vi "Begin.vi"(11 "Image Size":T1=enum."320x240") -> (0 "error out":errorcluster)   [LabVIEW 2013]
doc: "Called before other user functions, this VI is expected to open initial I/O refnums, load in file data, and do all program initialization. Notice that the <B>error out</B> terminal is simply used for data flow. Wiring it to other structures or subVIs ensures that this VI runs first."
uses:
  <vilib>/Rock Robotics/WPI/Camera/WPI_CameraImageSize.ctl
  <vilib>/Rock Robotics/WPI/DriverStation/WPI_DriverStationRobotMode2.ctl
  <vilib>/Rock Robotics/WPI/Joystick/WPI_JoystickDeviceEnum.ctl
  <vilib>/Rock Robotics/SystemInterfaces/DIO/FPGA_DIOPWMChannel.ctl
  <vilib>/Rock Robotics/SystemInterfaces/DIO/FPGA_DIORelayChannel.ctl
  <vilib>/Rock Robotics/SystemInterfaces/DIO/FPGA_DIOChannel.ctl
  <vilib>/Rock Robotics/SystemInterfaces/Typedef/FPGA_TypedefDigitalModule.ctl
  <vilib>/Rock Robotics/WPI/Solenoid/WPI_SolenoidChannel.ctl
  <vilib>/Rock Robotics/WPI/Encoder/WPI_EncoderType.ctl
  <vilib>/Rock Robotics/SystemInterfaces/Typedef/FPGA_TypedefAnalogModule.ctl
  <vilib>/Rock Robotics/SystemInterfaces/AI/FPGA_AIChannel.ctl
  RefnameEnum.ctl
  Sally_Dashboard_2014/DBNameEnum.ctl
  <vilib>/Rock Robotics/WPI/Solenoid/WPI_SolenoidValue.ctl
  <vilib>/Rock Robotics/WPI/SafetyOutput/WPI_SafetyOutputConfigMenu.ctl
  QueueInstruction.ctl
  SubsystemEnum.ctl
  ActionEnum.ctl
  TeleopData.ctl
  <vilib>/Rock Robotics/SystemInterfaces/CounterEncoderSourceConvertion/FPGA_CounterEncoderSourceConvertionLVSourceType.ctl
  <vilib>/Rock Robotics/SystemInterfaces/DIO/FPGA_DIODigitalSourceChannel.ctl
  <vilib>/Rock Robotics/SystemInterfaces/AnalogTrigger/FPGA_AnalogTriggerIndex.ctl
  <vilib>/Rock Robotics/SystemInterfaces/AnalogTrigger/FPGA_AnalogTriggerOutType.ctl
  Robot Global Data.vi
  <vilib>/Rock Robotics/WPI/RobotDrive/WPI_RobotDriveOpen2MotorWithTalon.vi
  <vilib>/Rock Robotics/WPI/MotorControl/WPI_MotorControlOpen Talon.vi
  <vilib>/Rock Robotics/WPI/Counter/WPI_CounterDigitalInputToDigitalSource.vi
  <vilib>/Rock Robotics/WPI/Solenoid/WPI_SolenoidOpenSingle.vi
  <vilib>/Rock Robotics/WPI/Solenoid/WPI_SolenoidSetEnum.vi
  <vilib>/Rock Robotics/WPI/MotorControl/WPI_MotorControlOpen Jaguar.vi
  <vilib>/Rock Robotics/WPI/Compressor/WPI_CompressorGetSetRefNum.vi
  <vilib>/Rock Robotics/WPI/Counter/WPI_CounterOpen UpDown Mode.vi
  <vilib>/Rock Robotics/WPI/Camera/WPI_CameraWhite Balance Values.ctl
  <vilib>/Rock Robotics/WPI/Camera/WPI_CameraExposure Values.ctl
  <vilib>/Rock Robotics/WPI/Camera/WPI_CameraFrameRate.ctl
  <vilib>/Rock Robotics/SystemInterfaces/AI/FPGA_AIGyroChannel.ctl
  <vilib>/Rock Robotics/SystemInterfaces/Typedef/FPGA_TypedefAnalogModuleForGyro.ctl
panel:
  in  "LowerLimit (v)":dbl=-1.0
  in  "UpperLimit (v)":dbl=1.0
  out "error out 2":errorcluster
  in  "Version String":string="TruongFramework 1.5.2"
  # "DON'T FORGET TO MAKE THIS DEFAULT"
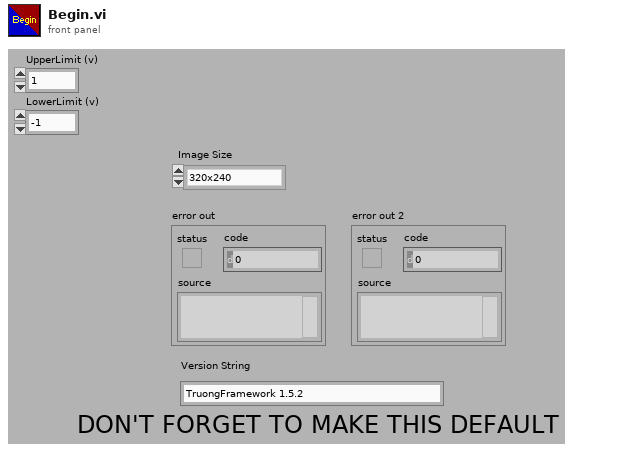
[diagram p1: front panel]
types:
  T1 = typedef "WPI_CameraImageSize.ctl" = enum16{"640x480", "320x240", "160x120"}
  T2 = typedef "TeleopData.ctl" = cluster{"cTankDriveLeft":dbl, "cTankDriveRight":dbl, "cHalfSpeed":bool, "cClimbWeight":bool, "cClimbStart":bool, "cRpmControl":dbl, "cAngleControl":dbl, "cQuickShoot":bool, "cLauncherWheel":bool, "cFirePneumatic":bool, "cPresetLow":bool, "cPresetHigh":bool, "cPresetClimbLow":bool, "cPresetClimbHigh":bool, "cLauncherAngle":bool, "cResetAngleEncoder":bool, "IDNum":i32, "TeleopInterval":i32}
  T3 = typedef "QueueInstruction.ctl" = cluster{"Data":variant, "Subsystem":T4, "Action":T5}
  T4 = typedef "SubsystemEnum.ctl" = enum16{"TankDrive", "FirePneumatic", "Climber", "ClimbWeight", "ShooterAngle"}
  T5 = typedef "ActionEnum.ctl" = enum16{"Init", "SetValue"}
  T6 = typedef "WPI_SafetyOutputConfigMenu.ctl" = enum16{"Enable", "Disable"}
  T7 = typedef "WPI_SolenoidValue.ctl" = enum16{"Off", "On", "Forward", "Reverse"}
  T8 = typedef "RefnameEnum.ctl" = enum16{"FireLauncher", "Climber", "Shield", "TankDrive", "DriveEncoderL", "DriveEncoderR", "LauncherMotorRPM", "LauncherEncoderAnalog", "LauncherEncoderRPM", "ShooterLS", "DriveAlignLSLeft", "DriveAlignLSRight", "ClimbingLS", "LauncherEncoderAngle", "LauncherMotorAngle", "Gamepad1", "Gamepad2", "Compressor", "ClimbWeightSol3", "ClimbWeightSol4"}
  T9 = typedef "WPI_SolenoidChannel.ctl" = enum8{"Solenoid 1", "Solenoid 2", "Solenoid 3", "Solenoid 4", "Solenoid 5", "Solenoid 6", "Solenoid 7", "Solenoid 8", "Invalid"}
  T10 = typedef "FPGA_DIOChannel.ctl" = enum8{"DIO 1", "DIO 2", "DIO 3", "DIO 4", "DIO 5", "DIO 6", "DIO 7", "DIO 8", "DIO 9", "DIO 10", "DIO 11", "DIO 12", "DIO 13", "DIO 14", "Invalid"}
  T11 = typedef "FPGA_TypedefDigitalModule.ctl" = enum16{"Digital Module 1", "Digital Module 2"}
  T12 = typedef "DBNameEnum.ctl" = enum16{"AutoInstructions", "DriveLoopTime", "DriveAlignLSLeft", "DriveAlignLSRight", "Use2DriveAlign", "ClimbLS", "LauncherAngleMatches", "FrameworkVersion", "sLauncherAngle", "LauncherTargetAngle", "sLauncherRPM", "LauncherTargetRPM", "sDriveDistance", "LauncherMotorValue", "PullbackTol", "FireTol", "LauncherRPMTol", "LauncherAngleTol", "InitialWait", "WaitBetweenLaunch", "AnglePresets", "RPMPresets", "UseAngleEncoder", "UseLauncherEncoder", "UseLauncherPID", "QSWaitBeforeFire", "QSWaitBeforeRetract", "AngleForwardValue", "AngleBackwardValue", "UseClusterArray", "BackupAuto", "ReverseDriveIndicate", "HalfSpeedFactor"}
  T13 = typedef "FPGA_AIChannel.ctl" = enum8{"AI 1", "AI 2", "AI 3", "AI 4", "AI 5", "AI 6", "AI 7", "AI 8", "Invalid"}
  T14 = typedef "FPGA_TypedefAnalogModule.ctl" = enum16{"Analog Module 1", "Analog Module 2"}
  T15 = typedef "WPI_EncoderType.ctl" = enum16{"1x", "2x", "4x"}
  T16 = typedef "FPGA_DIORelayChannel.ctl" = enum8{"Relay 1", "Relay 2", "Relay 3", "Relay 4", "Relay 5", "Relay 6", "Relay 7", "Relay 8", "Invalid"}
  T17 = typedef "FPGA_DIOPWMChannel.ctl" = enum8{"PWM 1", "PWM 2", "PWM 3", "PWM 4", "PWM 5", "PWM 6", "PWM 7", "PWM 8", "PWM 9", "PWM 10", "Invalid"}
  T18 = typedef "WPI_JoystickDeviceEnum.ctl" = enum16{"USB 1", "USB 2", "USB 3", "USB 4", "Kinect 1", "Kinect 2"}
  T19 = typedef "WPI_DriverStationRobotMode2.ctl" = enum16{"Autonomous Disabled", "Autonomous Enabled", "Teleop Disabled", "Teleop Enabled", "Timeout", "Finish", "Test Disabled", "Test Enabled"}
  T20 = enum16{"Rising Edge", "Falling Edge", "Raising & Falling Edge", "Disabled"}
  T21 = typedef "WPI_DigitalInputDevRef.ctl" = cluster{"DevStatus":errorcluster, "DIO Channel":T10, "Digital Module":T11}
  T22 = typedef "FPGA_CounterEncoderSourceConvertionLVSourceType.ctl" = cluster{"DevStatus":errorcluster, "AnalogTriggerMode?":bool, "DigitalMode":cluster{"Digital Module":T11, "DIO Channel":T23}, "AnalogTriggerMode":cluster{"AnalogTriggerIndex":T24, "OutputType":T25}}
  T23 = typedef "FPGA_DIODigitalSourceChannel.ctl" = enum8{"DIO 1", "DIO 2", "DIO 3", "DIO 4", "DIO 5", "DIO 6", "DIO 7", "DIO 8", "DIO 9", "DIO 10", "DIO 11", "DIO 12", "DIO 13", "DIO 14", "Disabled"}
  T24 = typedef "FPGA_AnalogTriggerIndex.ctl" = enum8{"Trig 0", "Trig 1", "Trig 2", "Trig 3", "Trig 4", "Trig 5", "Trig 6", "Trig 7", "Invalid"}
  T25 = typedef "FPGA_AnalogTriggerOutType.ctl" = enum16{"InWindow", "TriggerState", "Rising", "Falling"}
  T26 = typedef "WPI_EncoderDevRef.ctl" = cluster{"DevStatus":errorcluster, "EncoderIndex":T27, "CounterIndex":T28, "DistancePerCount":dbl, "Decoding Type":T15}
  T27 = typedef "FPGA_EncoderIdx.ctl" = enum8{"Enc 0", "Enc 1", "Enc 2", "Enc 3", "Invalid"}
  T28 = typedef "FPGA_CounterCtrSystemIndex.ctl" = enum8{"Ctr 0", "Ctr 1", "Ctr 2", "Ctr 3", "Ctr 4", "Ctr 5", "Ctr 6", "Ctr 7", "Invalid"}
  T29 = typedef "WPI_CounterDevRef.ctl" = cluster{"DevStatus":errorcluster, "CntIndex":T28}
  T30 = typedef "FPGA_AIGyroChannel.ctl" = enum8{"AI 1", "AI 2", "Invalid"}
  T31 = typedef "FPGA_TypedefAnalogModuleForGyro.ctl" = enum16{"Analog Module 1"}
  T32 = typedef "WPI_GyroDevRef.ctl" = cluster{"DevStatus":errorcluster, "Analog Module":T14, "Analog Channel":T13, "Offset":dbl, "Gain (VoltsPerDegree/Second)":dbl}
  T33 = typedef "WPI_MotorControlDeviceRef.ctl" = cluster{"DeviceStatus":errorcluster, "Type":enum16{"PWM", "CAN"}, "PWM":cluster{"Digital Module":T11, "PWM Channel":T17, "DeadBand":T34}, "CAN":cluster{"Device Number":u8, "Control Mode":T35, "Semaphore":T36, "Max Vout":dbl}, "Invert":bool, "TransformRef":T37, "InvTransformRef":T37}
  T34 = typedef "WPI_PWMDeadband.ctl" = cluster{"Name":string, "maxPositivePwm":i32, "minPositivePwm":i32, "centerPwm":i32, "maxNegativePwm":i32, "minNegativePwm":i32, "angularRange":u16}
  T35 = typedef "WPI_CANJaguar_ControlMode.ctl" = enum8{"Percent VBus", "Current", "Speed", "Position", "Voltage"}
  T36 = typedef "Semaphore RefNum" = refnum<k1>
  T37 = typedef "WPI_PWMTransform_ConPane.ctl" = refnum<vi>
  T38 = typedef "WPI_RelayDevRef.ctl" = cluster{"DevStatus":errorcluster, "Relay Channel":T16, "Digital Module":T11, "Relay Direction":T39}
  T39 = typedef "WPI_RelayDirection.ctl" = enum16{"Both directions", "Forward only", "Reverse only"}
  T40 = typedef "WPI_SolenoidDevRef.ctl" = cluster{"DevStatus":errorcluster, "Solenoid Module":T41, "Forward Solenoid Channel":T9, "Reverse Solenoid Channel":T9}
  T41 = typedef "FPGA_TypedefSolenoidModule.ctl" = enum16{"Solenoid Module 1", "Solenoid Module 2"}
  T42 = typedef "WPI_CompressorDevRef.ctl" = cluster{"DevStatus":errorcluster, "DigitalInputDevRef":T21, "RelayDevRef":T38}
  T43 = typedef "WPI_RobotDriveDevRef.ctl" = cluster{"DevStatus":errorcluster, "Motors[]":T33[], "Square Inputs":bool, "Max Output":dbl, "Isochronous":bool}
  T44 = typedef "WPI_CameraFrameRate.ctl" = u32
  T45 = typedef "WPI_CameraExposure Values.ctl" = enum16{"Auto", "Flicker-free 50 Hz", "Flicker-free 60 Hz", "Hold current"}
  T46 = typedef "WPI_CameraWhite Balance Values.ctl" = enum16{"Auto", "Fixed indoor", "Fixed outdoor 1", "Fixed outdoor 2", "Fixed fluorescent 1", "Fixed fluorescent 2", "Hold current"}
  T47 = typedef "WPI_CameraDevRef.ctl" = cluster{"Camera Address":string, "CameraStatus":errorcluster, "Acquire Image Notifier":refnum<notifier>}
  T48 = typedef "WPI_JoystickDevRef.ctl" = cluster{"Device":T18}
  T49 = typedef "WPI_AnalogChannelDevRef.ctl" = cluster{"DevStatus":errorcluster, "Analog Module":T14, "Analog Channel":T13}
  T50 = typedef "FPGA_AnalogTriggerDevRef.ctl" = cluster{"DevStatus":errorcluster, "AnalogTriggerIndex":T24}
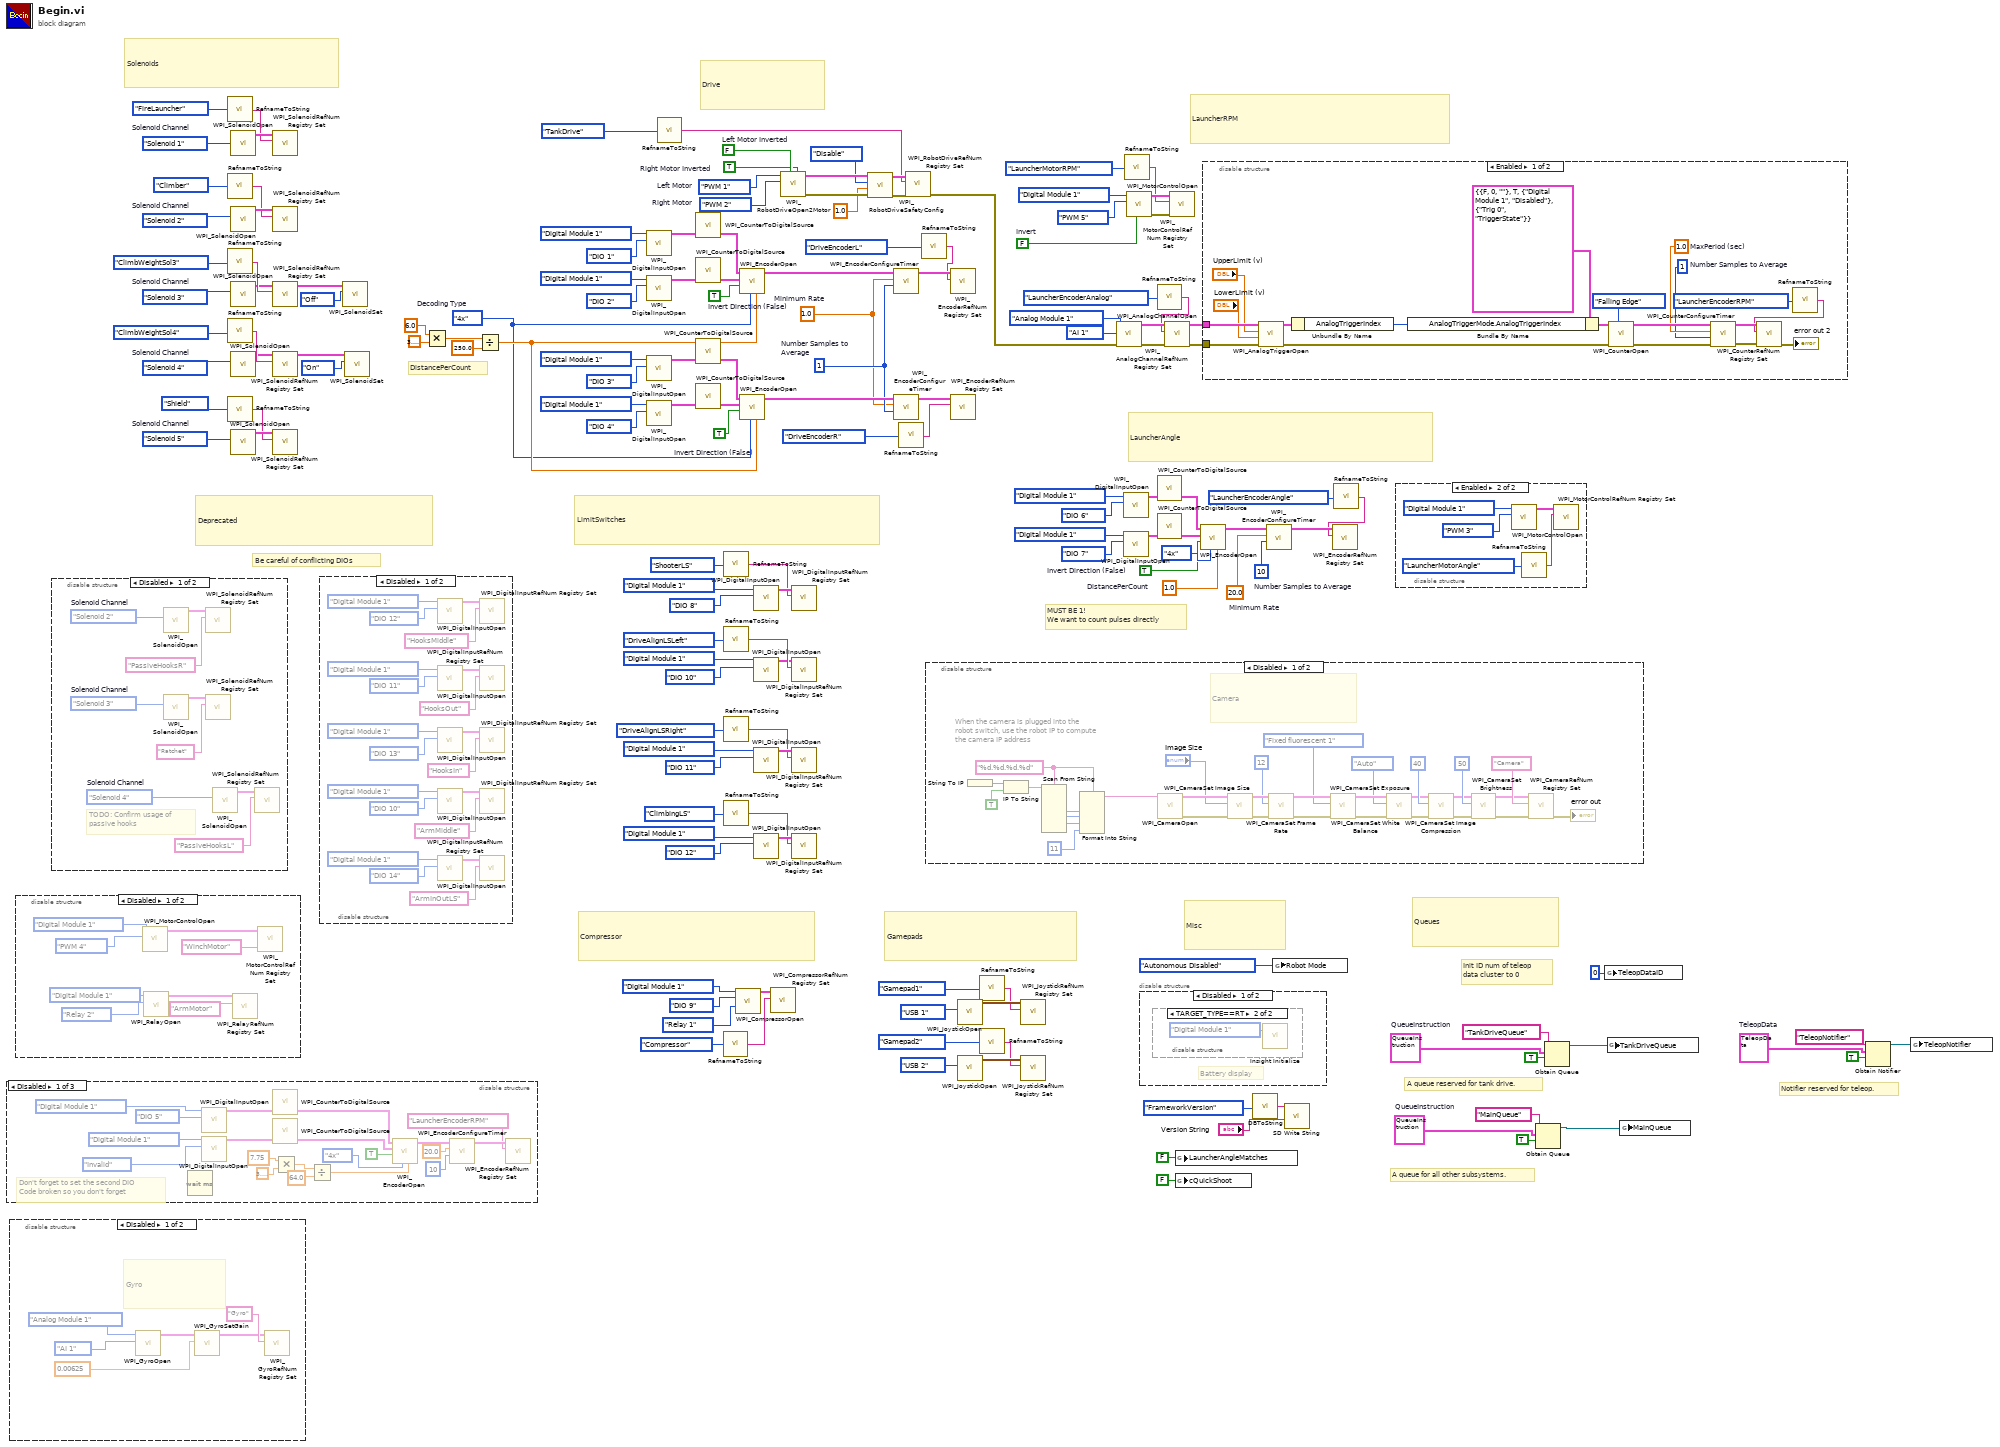
[diagram p0: block diagram]
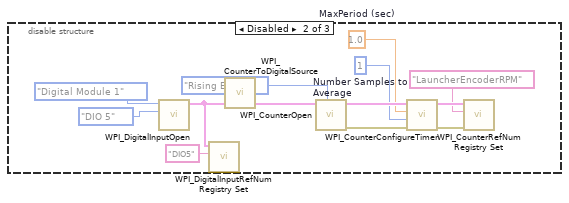
[diagram p8: hidden frame]
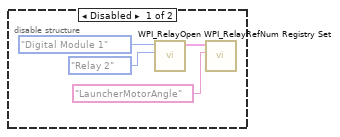
[diagram p12: hidden frame]
diagram:
  w5 = T2 {"cTankDriveLeft"=0.0, "cTankDriveRight"=0.0, "cHalfSpeed"=FALSE, "cClimbWeight"=FALSE, "cClimbStart"=FALSE, "cRpmControl"=0.0, "cAngleControl"=0.0, "cQuickShoot"=FALSE, "cLauncherWheel"=FALSE, "cFirePneumatic"=FALSE, "cPresetLow"=FALSE, "cPresetHigh"=FALSE, "cPresetClimbLow"=FALSE, "cPresetClimbHigh"=FALSE, "cLauncherAngle"=FALSE, "cResetAngleEncoder"=FALSE, "IDNum"=0, "TeleopInterval"=0}  # TeleopData
  w10 = T3 {"Data"=variant, "Subsystem"=enum."TankDrive", "Action"=enum."Init"}  # QueueInstruction
  w11 = T3 {"Data"=variant, "Subsystem"=enum."TankDrive", "Action"=enum."Init"}  # QueueInstruction
  w25 = WPI_SolenoidChannel."Solenoid 4"  # Solenoid Channel
  w29 = WPI_SolenoidChannel."Solenoid 3"  # Solenoid Channel
  w85 = 1.0  # DistancePerCount
  w88 = TRUE  # Invert Direction (False)
  w89 = TRUE  # Invert Direction (False)
  w93 = WPI_SolenoidChannel."Solenoid 5"  # Solenoid Channel
  w95 = WPI_SolenoidChannel."Solenoid 2"  # Solenoid Channel
  w100 = TRUE  # Invert Direction (False)
  w102 = u8 10  # Number Samples to Average
  w103 = 20.0  # Minimum Rate
  w115 = WPI_SolenoidChannel."Solenoid 1"  # Solenoid Channel
  w90 = WPI_EncoderType."4x"  # Decoding Type
  w87 = u8 1  # Number Samples to Average
  w86 = 1.0  # Minimum Rate
  w144 = FALSE  # Invert
  w148 = FPGA_DIOPWMChannel."PWM 2"  # Right Motor
  w149 = FPGA_DIOPWMChannel."PWM 1"  # Left Motor
  w150 = TRUE  # Right Motor Inverted
  w151 = FALSE  # Left Motor Inverted
  # "Init ID num of teleop\ndata cluster to 0"
  # "Notifier reserved for teleop."
  # "A queue reserved for tank drive."
  # "A queue for all other subsystems."
  # "Queues"
  # "Be careful of conflicting DIOs"
  # "DistancePerCount"
  # "Deprecated"
  # "LimitSwitches"
  # "Compressor"
  # "Solenoids"
  # "LauncherAngle"
  # "LauncherRPM"
  # "Misc"
  # "Gamepads"
  # "Drive"
  # "MUST BE 1!\nWe want to count pulses directly"
  n1 = disable-structure shown="Disabled" {
    frame Disabled {
      # "Don't forget to set the second DIO\nCode broken so you don't forget"
      n2 = Wait (ms)() -> ()  [unwired: 1 in, 1 out]
      n3 = call <vilib>:"WPI_DigitalInputOpen.vi"("DIO Channel"=FPGA_DIOChannel."DIO 5", "Digital Module (Module 1)"=FPGA_TypedefDigitalModule."Digital Module 1") -> ("DigitalInputDevRef"=w174:T21)  [unwired: 1 in, 8 out]
      n4 = call <vilib>:"WPI_DigitalInputOpen.vi"("DIO Channel"=FPGA_DIOChannel."Invalid", "Digital Module (Module 1)"=FPGA_TypedefDigitalModule."Digital Module 1") -> ("DigitalInputDevRef"=w175:T21)  [unwired: 1 in, 8 out]
      n5 = call-poly <vilib>:"WPI_CounterToDigitalSource.vi"("DigitalInputDevRef"=w174) -> ("Digital Source"=w173:T22)  [unwired: 6 out]
      n6 = call-poly <vilib>:"WPI_CounterToDigitalSource.vi"("DigitalInputDevRef"=w175) -> ("Digital Source"=w176:T22)  [unwired: 6 out]
      n7 = Multiply(x=7.75, y=3.141592653589793) -> (x*y=w158:dbl)
      n8 = Divide(x=w158, y=64.0) -> (x/y=w161:dbl)
      n9 = call <vilib>:"WPI_EncoderOpen.vi"("DistancePerCount"=w161, "Decoding Type"=WPI_EncoderType."4x", "Invert Direction (False)"=TRUE, "BSource"=w176, "ASource"=w173) -> ("EncoderDevRef"=w170:T26)  [unwired: 3 in, 3 out]
      n10 = call <vilib>:"WPI_EncoderConfigureTimer.vi"("Number Samples to Average"=u8 10, "Minimum Rate"=20.0, "EncoderDevRef"=w170) -> ("EncoderDevRef"=w167:T26)  [unwired: 1 in, 7 out]
      n11 = call <vilib>:"WPI_EncoderRefNum Registry Set.vi"("refnum name"="LauncherEncoderRPM", "EncoderDevRef"=w167) -> ()  [unwired: 8 in, 2 out]
    }
    frame Disabled {
      w187 = u8 1  # Number Samples to Average
      w188 = 1.0  # MaxPeriod (sec)
      n12 = call <vilib>:"WPI_DigitalInputOpen.vi"("DIO Channel"=FPGA_DIOChannel."DIO 5", "Digital Module (Module 1)"=FPGA_TypedefDigitalModule."Digital Module 1") -> ("DigitalInputDevRef"=w178:T21)  [unwired: 8 in, 1 out]
      n13 = call <vilib>:"WPI_DigitalInputRefNum Registry Set.vi"("refnum name"="DIO5", "DigitalInputDevRef"=w178) -> ()  [unwired: 8 in, 2 out]
      n14 = call-poly <vilib>:"WPI_CounterToDigitalSource.vi"("DigitalInputDevRef"=w178) -> ("Digital Source"=w181:T22)  [unwired: 6 out]
      n15 = call-poly <vilib>:"WPI_CounterOpen.vi"("UpEdge"=T20."Rising Edge", "Up Source"=w181) -> ("error out"=w183:errorcluster, "CounterDevRef"=w189:T29)  [unwired: 8 in]
      n16 = call <vilib>:"WPI_CounterConfigureTimer.vi"("error in (no error)"=w183, "Number Samples to Average"=w187, "MaxPeriod (sec)"=w188, "CounterDevRef in"=w189) -> ("error out"=w182:errorcluster, "CounterDevRef out"=w186:T29)  [unwired: 6 in]
      n17 = call <vilib>:"WPI_CounterRefNum Registry Set.vi"("error in (no error)"=w182, "refnum name"="LauncherEncoderRPM", "CounterDevRef"=w186) -> ()  [unwired: 7 in, 2 out]
    }
    frame Enabled {
      # "LauncherRPM Deprecated"
    }
  }
  n18 = disable-structure shown="Disabled" {
    frame Disabled {
      # "Gyro"
      n19 = call <vilib>:"WPI_GyroOpen.vi"("Analog Channel"=FPGA_AIGyroChannel."AI 1", "Analog Module (Module 1)"=FPGA_TypedefAnalogModuleForGyro."Analog Module 1") -> ("GyroDevRef"=w192:T32)  [unwired: 7 in, 2 out]
      n20 = call <vilib>:"WPI_GyroSetGain.vi"("Gain (VoltsPerDegree/Second)"=0.00625, "GyroDevRef"=w192) -> ("GyroDevRef"=w191:T32)  [unwired: 8 in, 1 out]
      n21 = call <vilib>:"WPI_GyroRefNum Registry Set.vi"("refnum name"="Gyro", "GyroDevRef"=w191) -> ()  [unwired: 8 in, 2 out]
    }
    frame Enabled {
    }
  }
  n22 = disable-structure shown="Disabled" {
    frame Disabled {
      n23 = call-poly <vilib>:"WPI_MotorControlOpen.vi"("PWM Channel"=FPGA_DIOPWMChannel."PWM 4", "Digital Module (Module 1)"=FPGA_TypedefDigitalModule."Digital Module 1") -> ("MotorControlDeviceRef"=w201:T33)  [unwired: 8 in, 1 out]
      n24 = call <vilib>:"WPI_RelayOpen.vi"("Relay Channel"=FPGA_DIORelayChannel."Relay 2", "Digital Module (Module 1)"=FPGA_TypedefDigitalModule."Digital Module 1") -> ("RelayDevRef"=w197:T38)  [unwired: 8 in, 1 out]
      n25 = call <vilib>:"WPI_RelayRefNum Registry Set.vi"("refnum name"="ArmMotor", "RelayDevRef"=w197) -> ()  [unwired: 8 in, 2 out]
      n26 = call <vilib>:"WPI_MotorControlRefNum Registry Set.vi"("refnum name"="WinchMotor", "MotorControlDevRef"=w201) -> ()  [unwired: 8 in, 2 out]
    }
    frame Enabled {
    }
  }
  n27 = disable-structure shown="Disabled" {
    frame Disabled {
      w206 = WPI_SolenoidChannel."Solenoid 2"  # Solenoid Channel
      w209 = WPI_SolenoidChannel."Solenoid 4"  # Solenoid Channel
      w212 = WPI_SolenoidChannel."Solenoid 3"  # Solenoid Channel
      # "TODO: Confirm usage of\npassive hooks"
      n28 = call-poly <vilib>:"WPI_SolenoidOpen.vi"("Solenoid Channel"=w206) -> ("SolenoidDevRef"=w205:T40)  [unwired: 2 in, 8 out]
      n29 = call-poly <vilib>:"WPI_SolenoidOpen.vi"("Solenoid Channel"=w212) -> ("SolenoidDevRef"=w211:T40)  [unwired: 2 in, 8 out]
      n30 = call <vilib>:"WPI_SolenoidRefNum Registry Set.vi"("refnum name"="PassiveHooksR", "SolenoidDevRef"=w205) -> ()  [unwired: 8 in, 2 out]
      n31 = call <vilib>:"WPI_SolenoidRefNum Registry Set.vi"("refnum name"="Ratchet", "SolenoidDevRef"=w211) -> ()  [unwired: 8 in, 2 out]
      n32 = call-poly <vilib>:"WPI_SolenoidOpen.vi"("Solenoid Channel"=w209) -> ("SolenoidDevRef"=w208:T40)  [unwired: 2 in, 8 out]
      n33 = call <vilib>:"WPI_SolenoidRefNum Registry Set.vi"("refnum name"="PassiveHooksL", "SolenoidDevRef"=w208) -> ()  [unwired: 8 in, 2 out]
    }
    frame Enabled {
    }
  }
  n34 = call "RefnameToString.vi"("Enum"=RefnameEnum."FireLauncher") -> ("Refname"=w68:string)
  n35 = call "RefnameToString.vi"("Enum"=RefnameEnum."Climber") -> ("Refname"=w66:string)
  n36 = call "RefnameToString.vi"("Enum"=RefnameEnum."ClimbWeightSol3") -> ("Refname"=w32:string)
  n37 = call "RefnameToString.vi"("Enum"=RefnameEnum."ClimbWeightSol4") -> ("Refname"=w28:string)
  n38 = call "RefnameToString.vi"("Enum"=RefnameEnum."Shield") -> ("Refname"=w64:string)
  n39 = call-poly <vilib>:"WPI_SolenoidOpen.vi"("Solenoid Channel"=w115) -> ("SolenoidDevRef"=w114:T40)  [unwired: 2 in, 8 out]
  n40 = call-poly <vilib>:"WPI_SolenoidOpen.vi"("Solenoid Channel"=w95) -> ("SolenoidDevRef"=w94:T40)  [unwired: 2 in, 8 out]
  n41 = call-poly <vilib>:"WPI_SolenoidOpen.vi"("Solenoid Channel"=w29) -> ("SolenoidDevRef"=w30:T40)  [unwired: 2 in, 8 out]
  n42 = call-poly <vilib>:"WPI_SolenoidOpen.vi"("Solenoid Channel"=w25) -> ("SolenoidDevRef"=w26:T40)  [unwired: 2 in, 8 out]
  n43 = call-poly <vilib>:"WPI_SolenoidOpen.vi"("Solenoid Channel"=w93) -> ("SolenoidDevRef"=w92:T40)  [unwired: 2 in, 8 out]
  n44 = call <vilib>:"WPI_SolenoidRefNum Registry Set.vi"("refnum name"=w68, "SolenoidDevRef"=w114) -> ()  [unwired: 8 in, 2 out]
  n45 = call <vilib>:"WPI_SolenoidRefNum Registry Set.vi"("refnum name"=w66, "SolenoidDevRef"=w94) -> ()  [unwired: 8 in, 2 out]
  n46 = call <vilib>:"WPI_SolenoidRefNum Registry Set.vi"("refnum name"=w32, "SolenoidDevRef"=w30) -> ("SolenoidDevRef"=w24:T40)  [unwired: 8 in, 1 out]
  n47 = call <vilib>:"WPI_SolenoidRefNum Registry Set.vi"("refnum name"=w28, "SolenoidDevRef"=w26) -> ("SolenoidDevRef"=w23:T40)  [unwired: 8 in, 1 out]
  n48 = call <vilib>:"WPI_SolenoidRefNum Registry Set.vi"("refnum name"=w64, "SolenoidDevRef"=w92) -> ()  [unwired: 8 in, 2 out]
  n49 = disable-structure shown="Disabled" {
    frame Disabled {
      n50 = call <vilib>:"WPI_DigitalInputOpen.vi"("DIO Channel"=FPGA_DIOChannel."DIO 12", "Digital Module (Module 1)"=FPGA_TypedefDigitalModule."Digital Module 1") -> ("DigitalInputDevRef"=w216:T21)  [unwired: 8 in, 1 out]
      n51 = call <vilib>:"WPI_DigitalInputOpen.vi"("DIO Channel"=FPGA_DIOChannel."DIO 11", "Digital Module (Module 1)"=FPGA_TypedefDigitalModule."Digital Module 1") -> ("DigitalInputDevRef"=w220:T21)  [unwired: 8 in, 1 out]
      n52 = call <vilib>:"WPI_DigitalInputOpen.vi"("DIO Channel"=FPGA_DIOChannel."DIO 13", "Digital Module (Module 1)"=FPGA_TypedefDigitalModule."Digital Module 1") -> ("DigitalInputDevRef"=w224:T21)  [unwired: 8 in, 1 out]
      n53 = call <vilib>:"WPI_DigitalInputOpen.vi"("DIO Channel"=FPGA_DIOChannel."DIO 10", "Digital Module (Module 1)"=FPGA_TypedefDigitalModule."Digital Module 1") -> ("DigitalInputDevRef"=w228:T21)  [unwired: 8 in, 1 out]
      n54 = call <vilib>:"WPI_DigitalInputOpen.vi"("DIO Channel"=FPGA_DIOChannel."DIO 14", "Digital Module (Module 1)"=FPGA_TypedefDigitalModule."Digital Module 1") -> ("DigitalInputDevRef"=w232:T21)  [unwired: 8 in, 1 out]
      n55 = call <vilib>:"WPI_DigitalInputRefNum Registry Set.vi"("refnum name"="HooksMiddle", "DigitalInputDevRef"=w216) -> ()  [unwired: 8 in, 2 out]
      n56 = call <vilib>:"WPI_DigitalInputRefNum Registry Set.vi"("refnum name"="HooksOut", "DigitalInputDevRef"=w220) -> ()  [unwired: 8 in, 2 out]
      n57 = call <vilib>:"WPI_DigitalInputRefNum Registry Set.vi"("refnum name"="HooksIn", "DigitalInputDevRef"=w224) -> ()  [unwired: 8 in, 2 out]
      n58 = call <vilib>:"WPI_DigitalInputRefNum Registry Set.vi"("refnum name"="ArmMiddle", "DigitalInputDevRef"=w228) -> ()  [unwired: 8 in, 2 out]
      n59 = call <vilib>:"WPI_DigitalInputRefNum Registry Set.vi"("refnum name"="ArmInOutLS", "DigitalInputDevRef"=w232) -> ()  [unwired: 8 in, 2 out]
    }
    frame Enabled {
    }
  }
  n60 = call-poly <vilib>:"WPI_SolenoidSet.vi"("Value"=WPI_SolenoidValue."Off", "SolenoidDevRef"=w24) -> ()  [unwired: 8 in, 2 out]
  n61 = call-poly <vilib>:"WPI_SolenoidSet.vi"("Value"=WPI_SolenoidValue."On", "SolenoidDevRef"=w23) -> ()  [unwired: 8 in, 2 out]
  n62 = Multiply(x=6.0, y=3.141592653589793) -> (x*y=w97:dbl)
  n63 = Divide(x=w97, y=250.0) -> (x/y=w91:dbl)
  n64 = call <vilib>:"WPI_DigitalInputOpen.vi"("DIO Channel"=FPGA_DIOChannel."DIO 1", "Digital Module (Module 1)"=FPGA_TypedefDigitalModule."Digital Module 1") -> ("DigitalInputDevRef"=w136:T21)  [unwired: 1 in, 8 out]
  n65 = call <vilib>:"WPI_DigitalInputOpen.vi"("DIO Channel"=FPGA_DIOChannel."DIO 2", "Digital Module (Module 1)"=FPGA_TypedefDigitalModule."Digital Module 1") -> ("DigitalInputDevRef"=w137:T21)  [unwired: 1 in, 8 out]
  n66 = call <vilib>:"WPI_DigitalInputOpen.vi"("DIO Channel"=FPGA_DIOChannel."DIO 3", "Digital Module (Module 1)"=FPGA_TypedefDigitalModule."Digital Module 1") -> ("DigitalInputDevRef"=w123:T21)  [unwired: 1 in, 8 out]
  n67 = call <vilib>:"WPI_DigitalInputOpen.vi"("DIO Channel"=FPGA_DIOChannel."DIO 4", "Digital Module (Module 1)"=FPGA_TypedefDigitalModule."Digital Module 1") -> ("DigitalInputDevRef"=w124:T21)  [unwired: 1 in, 8 out]
  n68 = call "RefnameToString.vi"("Enum"=RefnameEnum."TankDrive") -> ("Refname"=w16:string)
  n69 = call-poly <vilib>:"WPI_CounterToDigitalSource.vi"("DigitalInputDevRef"=w136) -> ("Digital Source"=w135:T22)  [unwired: 6 out]
  n70 = call-poly <vilib>:"WPI_CounterToDigitalSource.vi"("DigitalInputDevRef"=w137) -> ("Digital Source"=w138:T22)  [unwired: 6 out]
  n71 = call-poly <vilib>:"WPI_CounterToDigitalSource.vi"("DigitalInputDevRef"=w123) -> ("Digital Source"=w122:T22)  [unwired: 6 out]
  n72 = call-poly <vilib>:"WPI_CounterToDigitalSource.vi"("DigitalInputDevRef"=w124) -> ("Digital Source"=w125:T22)  [unwired: 6 out]
  n73 = call "RefnameToString.vi"("Enum"=RefnameEnum."Compressor") -> ("Refname"=w45:string)
  n74 = call "RefnameToString.vi"("Enum"=RefnameEnum."ShooterLS") -> ("Refname"=w51:string)
  n75 = call "RefnameToString.vi"("Enum"=RefnameEnum."DriveAlignLSLeft") -> ("Refname"=w38:string)
  n76 = call "RefnameToString.vi"("Enum"=RefnameEnum."DriveAlignLSRight") -> ("Refname"=w49:string)
  n77 = call "RefnameToString.vi"("Enum"=RefnameEnum."ClimbingLS") -> ("Refname"=w47:string)
  n78 = call <vilib>:"WPI_CompressorOpen.vi"("Pressure Switch Digital Module (Module 1)"=FPGA_TypedefDigitalModule."Digital Module 1" ("Pressure Switch\nand Relay Module"), "Pressure Switch DIO Channel"=FPGA_DIOChannel."DIO 9" ("Pressure Switch Channel"), "Relay Channel"=FPGA_DIORelayChannel."Relay 1") -> ("CompressorDevRef"=w139:T42)  [unwired: 2 in, 10 out]
  n79 = call <vilib>:"WPI_EncoderOpen.vi"("DistancePerCount"=w91, "Decoding Type"=w90, "Invert Direction (False)"=w89, "BSource"=w138, "ASource"=w135) -> ("EncoderDevRef"=w132:T26)  [unwired: 3 in, 3 out]
  n80 = call <vilib>:"WPI_EncoderOpen.vi"("DistancePerCount"=w91, "Decoding Type"=w90, "Invert Direction (False)"=w88, "BSource"=w125, "ASource"=w122) -> ("EncoderDevRef"=w119:T26)  [unwired: 3 in, 3 out]
  n81 = call <vilib>:"WPI_DigitalInputOpen.vi"("DIO Channel"=FPGA_DIOChannel."DIO 8", "Digital Module (Module 1)"=FPGA_TypedefDigitalModule."Digital Module 1") -> ("DigitalInputDevRef"=w128:T21)  [unwired: 8 in, 1 out]
  n82 = call <vilib>:"WPI_DigitalInputOpen.vi"("DIO Channel"=FPGA_DIOChannel."DIO 10", "Digital Module (Module 1)"=FPGA_TypedefDigitalModule."Digital Module 1") -> ("DigitalInputDevRef"=w34:T21)  [unwired: 8 in, 1 out]
  n83 = call <vilib>:"WPI_DigitalInputOpen.vi"("DIO Channel"=FPGA_DIOChannel."DIO 11", "Digital Module (Module 1)"=FPGA_TypedefDigitalModule."Digital Module 1") -> ("DigitalInputDevRef"=w78:T21)  [unwired: 8 in, 1 out]
  n84 = call <vilib>:"WPI_DigitalInputOpen.vi"("DIO Channel"=FPGA_DIOChannel."DIO 12", "Digital Module (Module 1)"=FPGA_TypedefDigitalModule."Digital Module 1") -> ("DigitalInputDevRef"=w72:T21)  [unwired: 8 in, 1 out]
  n85 = call <vilib>:"WPI_CompressorRefNum Registry Set.vi"("refnum name"=w45, "CompressorDevRef"=w139) -> ()  [unwired: 8 in, 2 out]
  n86 = call-poly <vilib>:"WPI_RobotDriveOpen2Motor.vi"("Right Motor Inverted"=w150, "Left Motor Inverted"=w151, "Right Motor"=w148, "Left Motor"=w149) -> ("error out"=w17:errorcluster, "RobotDriveDevRef"=w20:T43)  [unwired: 6 in]
  n87 = call <vilib>:"WPI_DigitalInputRefNum Registry Set.vi"("refnum name"=w51, "DigitalInputDevRef"=w128) -> ()  [unwired: 8 in, 2 out]
  n88 = call <vilib>:"WPI_DigitalInputRefNum Registry Set.vi"("refnum name"=w38, "DigitalInputDevRef"=w34) -> ()  [unwired: 8 in, 2 out]
  n89 = call <vilib>:"WPI_DigitalInputRefNum Registry Set.vi"("refnum name"=w49, "DigitalInputDevRef"=w78) -> ()  [unwired: 8 in, 2 out]
  n90 = call <vilib>:"WPI_DigitalInputRefNum Registry Set.vi"("refnum name"=w47, "DigitalInputDevRef"=w72) -> ()  [unwired: 8 in, 2 out]
  n91 = call <vilib>:"WPI_RobotDriveSafetyConfig.vi"("error in (no error)"=w17, "timeout (s)"=1.0, "mode"=WPI_SafetyOutputConfigMenu."Disable", "RobotDriveDevRef"=w20) -> ("error out"=w18:errorcluster, "RobotDriveDevRef"=w19:T43)  [unwired: 6 in]
  n92 = call <vilib>:"WPI_EncoderConfigureTimer.vi"("Number Samples to Average"=w87, "Minimum Rate"=w86, "EncoderDevRef"=w132) -> ("EncoderDevRef"=w129:T26)  [unwired: 1 in, 7 out]
  n93 = call <vilib>:"WPI_EncoderConfigureTimer.vi"("Number Samples to Average"=w87, "Minimum Rate"=w86, "EncoderDevRef"=w119) -> ("EncoderDevRef"=w116:T26)  [unwired: 1 in, 7 out]
  n94 = call "RefnameToString.vi"("Enum"=RefnameEnum."DriveEncoderR") -> ("Refname"=w59:string)
  n95 = call <vilib>:"WPI_RobotDriveRefNum Registry Set.vi"("error in (no error)"=w18, "refnum name"=w16, "RobotDriveDevRef"=w19) -> ("error out"=w75:errorcluster)  [unwired: 7 in, 1 out]
  n96 = call "RefnameToString.vi"("Enum"=RefnameEnum."DriveEncoderL") -> ("Refname"=w61:string)
  n97 = disable-structure shown="Disabled" {
    frame Disabled {
      w235 = "%d.%d.%d.%d" ("format string")
      # "Camera"
      # "When the camera is plugged into the\nrobot switch, use the robot IP to compute\nthe camera IP address"
      n98 = String To IP() -> (0:w242:u32)  [unwired: 1 in]
      n99 = IP To String(1:TRUE ("dot notation? (F)"), 2:w242) -> (0:w240:string)
      n100 = Scan From String(format string=w235, input string=w240) -> (output 1=w239:i32, output 2=w238:i32, output 3=w237:i32)  [unwired: 7 in, 3 out]
      n101 = Format Into String(format string=w235, w239, w238, w237, 11 ("Compression")) -> (resulting string=w234:string)  [unwired: 2 in, 1 out]
      n102 = call <vilib>:"WPI_CameraOpen.vi"("Camera Address"=w234) -> ("error out"=w254:errorcluster, "CameraDevRef"=w255:T47)  [unwired: 1 in, 8 out]
      n103 = call <vilib>:"WPI_CameraSet Image Size.vi"("error in (no error)"=w254, "Image Size"="Image Size", "CameraDevRef"=w255) -> ("error out"=w253:errorcluster, "CameraDevRef Out"=w256:T47)  [unwired: 7 out]
      n104 = call <vilib>:"WPI_CameraSet Frame Rate.vi"("error in (no error)"=w253, "Frame Rate (fps)"=T44 12, "CameraDevRef"=w256) -> ("error out"=w252:errorcluster, "CameraDevRef Out"=w258:T47)  [unwired: 7 out]
      n105 = call <vilib>:"WPI_CameraSet White Balance.vi"("error in (no error)"=w252, "White Balance"=WPI_CameraWhite_Balance_Values."Fixed fluorescent 1", "CameraDevRef"=w258) -> ("error out"=w251:errorcluster, "CameraDevRef Out"=w257:T47)  [unwired: 7 out]
      n106 = call <vilib>:"WPI_CameraSet Exposure.vi"("error in (no error)"=w251, "Exposure"=WPI_CameraExposure_Values."Auto", "CameraDevRef"=w257) -> ("error out"=w250:errorcluster, "CameraDevRef Out"=w260:T47)  [unwired: 7 out]
      n107 = call <vilib>:"WPI_CameraSet Image Compression.vi"("error in (no error)"=w250, "Compression"=40, "CameraDevRef"=w260) -> ("error out"=w249:errorcluster, "CameraDevRef Out"=w259:T47)  [unwired: 7 out]
      n108 = call <vilib>:"WPI_CameraSet Brightness.vi"("error in (no error)"=w249, "Brightness"=50, "CameraDevRef"=w259) -> ("error out"=w247:errorcluster, "CameraDevRef Out"=w248:T47)  [unwired: 7 out]
      n109 = call <vilib>:"WPI_CameraRefNum Registry Set.vi"("error in (no error)"=w247, "refnum name"="Camera", "CameraDevRef"=w248) -> ("error out"=→"error out":errorcluster)  [unwired: 8 out]
    }
    frame Enabled {
    }
  }
  n110 = call <vilib>:"WPI_EncoderRefNum Registry Set.vi"("refnum name"=w61, "EncoderDevRef"=w129) -> ()  [unwired: 8 in, 2 out]
  n111 = call <vilib>:"WPI_EncoderRefNum Registry Set.vi"("refnum name"=w59, "EncoderDevRef"=w116) -> ()  [unwired: 8 in, 2 out]
  n112 = call <vilib>:"WPI_JoystickOpen.vi"("JoystickDevice"=WPI_JoystickDeviceEnum."USB 1") -> ("JoystickDevRef"=w155:T48)  [unwired: 10 in]
  n113 = call <vilib>:"WPI_JoystickOpen.vi"("JoystickDevice"=WPI_JoystickDeviceEnum."USB 2") -> ("JoystickDevRef"=w152:T48)  [unwired: 10 in]
  n114 = call "RefnameToString.vi"("Enum"=RefnameEnum."Gamepad1") -> ("Refname"=w41:string)
  n115 = call "RefnameToString.vi"("Enum"=RefnameEnum."Gamepad2") -> ("Refname"=w43:string)
  n116 = call <vilib>:"WPI_JoystickRefNum Registry Set.vi"("refnum name"=w41, "JoystickDevRef"=w155) -> ()  [unwired: 8 in, 2 out]
  n117 = call <vilib>:"WPI_JoystickRefNum Registry Set.vi"("refnum name"=w43, "JoystickDevRef"=w152) -> ()  [unwired: 8 in, 2 out]
  n118 = call <vilib>:"WPI_AnalogChannelOpen.vi"("error in (no error)"=w75, "Analog Channel"=FPGA_AIChannel."AI 1", "Analog Module (Module 1)"=FPGA_TypedefAnalogModule."Analog Module 1") -> ("error out"=w80:errorcluster, "AIDeviceRef"=w79:T49)  [unwired: 7 in]
  n119 = call <vilib>:"WPI_DigitalInputOpen.vi"("DIO Channel"=FPGA_DIOChannel."DIO 6", "Digital Module (Module 1)"=FPGA_TypedefDigitalModule."Digital Module 1") -> ("DigitalInputDevRef"=w111:T21)  [unwired: 1 in, 8 out]
  n120 = call <vilib>:"WPI_DigitalInputOpen.vi"("DIO Channel"=FPGA_DIOChannel."DIO 7", "Digital Module (Module 1)"=FPGA_TypedefDigitalModule."Digital Module 1") -> ("DigitalInputDevRef"=w112:T21)  [unwired: 1 in, 8 out]
  n121 = call "RefnameToString.vi"("Enum"=RefnameEnum."LauncherMotorRPM") -> ("Refname"=w57:string)
  n122 = call-poly <vilib>:"WPI_MotorControlOpen.vi"("Invert"=w144, "PWM Channel"=FPGA_DIOPWMChannel."PWM 5", "Digital Module (Module 1)"=FPGA_TypedefDigitalModule."Digital Module 1") -> ("error out"=w143:errorcluster, "MotorControlDeviceRef"=w147:T33)  [unwired: 7 in]
  n123 = disable-structure shown="Disabled" {
    frame Disabled {
      # "Battery display"
      n124 = disable-structure shown="TARGET_TYPE==RT" {
        frame condition #0 {
        }
        frame condition #1 (active) {
          n125 = call "Insight Initialize.vi"("Digital Module"=FPGA_TypedefDigitalModule."Digital Module 1") -> ()  [unwired: 2 in]
        }
      }
    }
    frame Enabled {
    }
  }
  n126 = call "RefnameToString.vi"("Enum"=RefnameEnum."LauncherEncoderAnalog") -> ("Refname"=w55:string)
  n127 = call-poly <vilib>:"WPI_CounterToDigitalSource.vi"("DigitalInputDevRef"=w111) -> ("Digital Source"=w110:T22)  [unwired: 6 out]
  n128 = call-poly <vilib>:"WPI_CounterToDigitalSource.vi"("DigitalInputDevRef"=w112) -> ("Digital Source"=w113:T22)  [unwired: 6 out]
  n129 = call <vilib>:"WPI_AnalogChannelRefNum Registry Set.vi"("error in (no error)"=w80, "refnum name"=w55, "AIDeviceRef"=w79) -> ("error out"=w73:errorcluster, "AIDeviceRef"=w74:T49)  [unwired: 7 in]
  n130 = call <vilib>:"WPI_MotorControlRefNum Registry Set.vi"("error in (no error)"=w143, "refnum name"=w57, "MotorControlDevRef"=w147) -> ()  [unwired: 7 in, 2 out]
  n131 = global write "Robot Global Data.vi" "LauncherAngleMatches"(FALSE) -> ()
  n132 = global write "Robot Global Data.vi" "cQuickShoot"(FALSE) -> ()
  n133 = call <vilib>:"WPI_EncoderOpen.vi"("DistancePerCount"=w85, "Decoding Type"=WPI_EncoderType."4x", "Invert Direction (False)"=w100, "BSource"=w113, "ASource"=w110) -> ("EncoderDevRef"=w107:T26)  [unwired: 3 in, 3 out]
  n134 = disable-structure shown="Enabled" {
    disable-tunnel: w74 -> [w270 _]
    disable-tunnel: w73 -> [w269 _]
    frame Enabled {
      w279 = u8 1  # Number Samples to Average
      w280 = 1.0  # MaxPeriod (sec)
      n135 = call <vilib>:"WPI_AnalogTriggerOpen.vi"("error in (no error)"=w269, "LowerLimit (v)"="LowerLimit (v)", "UpperLimit (v)"="UpperLimit (v)", "AnalogTriggerSource"=w270) -> ("error out"=w283:errorcluster, "AnalogTriggerDevRef"=w278:T50)  [unwired: 6 in]
      n136 = Unbundle By Name(w278) -> ("AnalogTriggerIndex"=w277:T24)
      n137 = Bundle By Name(cluster=T22 {"DevStatus"={"status"=FALSE, "code"=0, "source"=""}, "AnalogTriggerMode?"=TRUE, "DigitalMode"={"Digital Module"=enum."Digital Module 1", "DIO Channel"=enum."Disabled"}, "AnalogTriggerMode"={"AnalogTriggerIndex"=enum."Trig 0", "OutputType"=enum."TriggerState"}} ("Source"), "AnalogTriggerMode.AnalogTriggerIndex"=w277) -> (w275:T22)
      n138 = call-poly <vilib>:"WPI_CounterOpen.vi"("UpEdge"=T20."Falling Edge" ("UpEdge 1"), "error in (no error)"=w283, "Up Source"=w275) -> ("error out"=w281:errorcluster, "CounterDevRef"=w282:T29)  [unwired: 7 in]
      n139 = call <vilib>:"WPI_CounterConfigureTimer.vi"("error in (no error)"=w281, "Number Samples to Average"=w279, "MaxPeriod (sec)"=w280, "CounterDevRef in"=w282) -> ("error out"=w272:errorcluster, "CounterDevRef out"=w273:T29)  [unwired: 6 in]
      n140 = call "RefnameToString.vi"("Enum"=RefnameEnum."LauncherEncoderRPM") -> ("Refname"=w267:string)
      n141 = call <vilib>:"WPI_CounterRefNum Registry Set.vi"("error in (no error)"=w272, "refnum name"=w267, "CounterDevRef"=w273) -> ("error out"=→"error out 2":errorcluster)  [unwired: 7 in, 1 out]
    }
    frame Disabled {
    }
  }
  n142 = call "DBToString.vi"("Enum"=DBNameEnum."FrameworkVersion") -> ("Refname"=w39:string)
  n143 = call <vilib>:"WPI_EncoderConfigureTimer.vi"("Number Samples to Average"=w102, "Minimum Rate"=w103, "EncoderDevRef"=w107) -> ("EncoderDevRef"=w104:T26)  [unwired: 1 in, 7 out]
  n144 = global write "Robot Global Data.vi" "Robot Mode"(WPI_DriverStationRobotMode2."Autonomous Disabled" ("Robot Mode")) -> ()
  n145 = call <vilib>:"SD Write String.vi"("String"="Version String", "Name"=w39) -> ()  [unwired: 8 in, 2 out]
  n146 = call "RefnameToString.vi"("Enum"=RefnameEnum."LauncherEncoderAngle") -> ("Refname"=w53:string)
  n147 = call <vilib>:"WPI_EncoderRefNum Registry Set.vi"("refnum name"=w53, "EncoderDevRef"=w104) -> ()  [unwired: 8 in, 2 out]
  n148 = disable-structure shown="Enabled" {
    frame Disabled {
      n149 = call <vilib>:"WPI_RelayOpen.vi"("Relay Channel"=FPGA_DIORelayChannel."Relay 2", "Digital Module (Module 1)"=FPGA_TypedefDigitalModule."Digital Module 1") -> ("RelayDevRef"=w285:T38)  [unwired: 8 in, 1 out]
      n150 = call <vilib>:"WPI_RelayRefNum Registry Set.vi"("refnum name"="LauncherMotorAngle", "RelayDevRef"=w285) -> ()  [unwired: 8 in, 2 out]
    }
    frame Enabled {
      n151 = call-poly <vilib>:"WPI_MotorControlOpen.vi"("PWM Channel"=FPGA_DIOPWMChannel."PWM 3", "Digital Module (Module 1)"=FPGA_TypedefDigitalModule."Digital Module 1") -> ("MotorControlDeviceRef"=w291:T33)  [unwired: 8 in, 1 out]
      n152 = call "RefnameToString.vi"("Enum"=RefnameEnum."LauncherMotorAngle") -> ("Refname"=w288:string)
      n153 = call <vilib>:"WPI_MotorControlRefNum Registry Set.vi"("refnum name"=w288, "MotorControlDevRef"=w291) -> ()  [unwired: 8 in, 2 out]
    }
  }
  n154 = Obtain Queue(name (unnamed)="MainQueue", element data type=w10, create if not found? (T)=TRUE) -> (queue out=w3:refnum<queue>)  [unwired: 2 in, 2 out]
  n155 = Obtain Queue(name (unnamed)="TankDriveQueue", element data type=w11, create if not found? (T)=TRUE) -> (queue out=w4:refnum<queue>)  [unwired: 2 in, 2 out]
  n156 = global write "Robot Global Data.vi" "TeleopDataID"(0 ("TeleopDataID")) -> ()
  n157 = global write "Robot Global Data.vi" "TankDriveQueue"(w4) -> ()
  n158 = global write "Robot Global Data.vi" "MainQueue"(w3) -> ()
  n159 = Obtain Notifier(name (unnamed)="TeleopNotifier", notification data type=w5, create if not found? (T)=TRUE) -> (notifier out=w2:refnum<notifier>)  [unwired: 1 in, 2 out]
  n160 = global write "Robot Global Data.vi" "TeleopNotifier"(w2) -> ()
